vi "globalTearDown.vi"(8 "error in (no error)":errorcluster, 11 "Logging Loopback in":refnum<class "Logging Loopback.lvclass">) -> (0 "error out":errorcluster, 3 "Logging Loopback out":refnum<class "Logging Loopback.lvclass">)   [LabVIEW 2020, in "Logging Loopback.lvclass"]
uses:
  Logging Loopback.lvclass
  Loopback/Loopback.lvclass
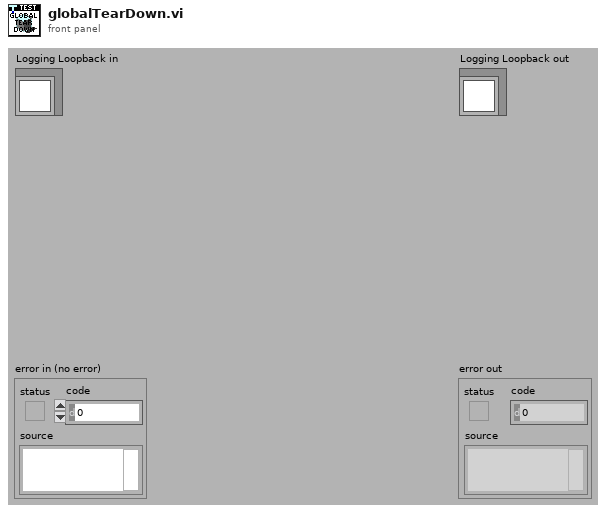
[diagram p1: front panel]
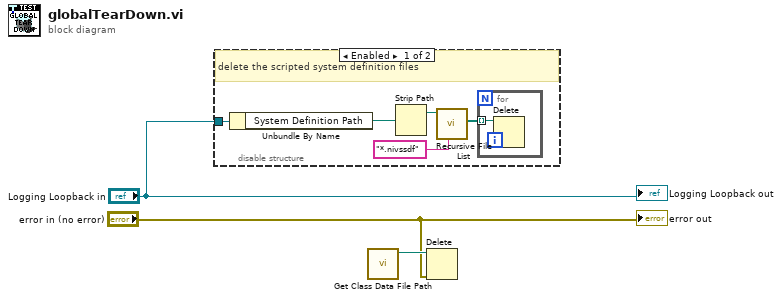
[diagram p0: block diagram]
diagram:
  n1 = disable-structure shown="Enabled" {
    disable-tunnel: "Logging Loopback in" -> [w8 _]
    frame Enabled {
      # "delete the scripted system definition files"
      n2 = Unbundle By Name(w8) -> ("System Definition Path"=w5:path)
      n3 = Strip Path(path=w5) -> (stripped path=w4:path)  [unwired: 1 out]
      n4 = call <vilib>:"Recursive File List.vi"("pattern"="*.nivssdf", "Folder Path"=w4) -> ("All Files in Dir"=w6:path[])  [unwired: 5 in, 4 out]
      n5 = for {
        tunnel: w6 -> [w9] mode=indexing
        n6 = Delete(path (use dialog)=w9) -> ()  [unwired: 4 in, 3 out]
      }
    }
    frame Disabled {
    }
  }
  n7 = call "Get Class Data File Path.vi"() -> ("Class Data File Path"=w3:path)  [unwired: 11 in]
  n8 = Delete(path (use dialog)=w3, error in="error in (no error)") -> ()  [unwired: 3 in, 3 out]
  "error out" <- "error in (no error)"
  "Logging Loopback out" <- "Logging Loopback in"
